vi "findNodes.vi"(0 "reference":refnum<class "Graph.lvclass">, 1 "bounds":T1 {"height" format="%.2f"; "width" format="%.2f"; "y" format="%.2f"; "x" format="%.2f"}, 5 "error in (no error)":errorcluster) -> (14 "reference out":refnum<class "Graph.lvclass">, 15 "FirstNode":refnum<class "AbstractNode.lvclass">, 16 "Nodes":refnum<class "AbstractNode.lvclass">[](array[class]), 17 "AnyFound":bool, 19 "error out":errorcluster)   [LabVIEW 2014, in "Graph.lvclass"]
doc: "Finds a node containing the given point.\n @param p a point\n @return a node containing p or null if no nodes contain p\n */\n public Node findNode(Point2D p)"
uses:
  <resource>/Framework/Providers/Open_GDS/UML/Graph_class/Graph.lvclass
  <resource>/Framework/Providers/Open_GDS/UML/General/Rectangle/Rectangle Rectangle2D.ctl
  <resource>/Framework/Providers/Open_GDS/UML/AbstractNode_class/AbstractNode.lvclass
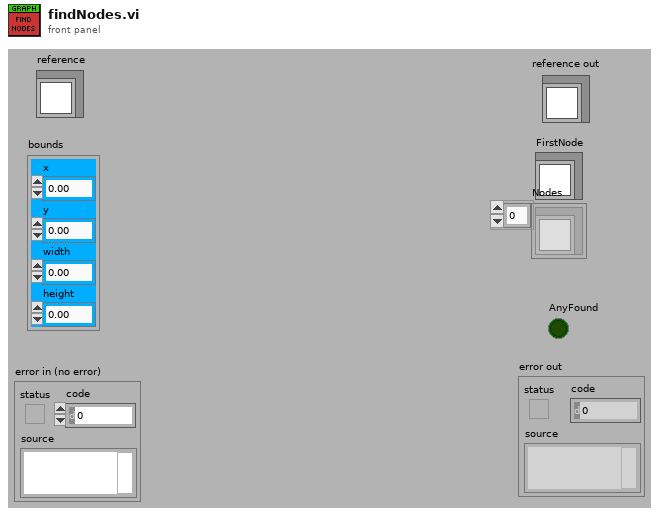
[diagram p1: front panel]
types:
  T1 = typedef "Rectangle Rectangle2D.ctl" = cluster{"x":dbl, "y":dbl, "width":dbl, "height":dbl}
  T2 = typedef "Graph.lvclass/ObjectAttributes.ctl" = cluster{"nodes":refnum<class "AbstractNode.lvclass">[], "edges":refnum<class "AbstractEdge.lvclass">[], "nodesToBeRemoved":refnum<class "AbstractNode.lvclass">[], "edgesToBeRemoved":refnum<class "AbstractEdge.lvclass">[], "needsLayout":bool, "LayoutNodes":refnum<class "AbstractNode.lvclass">[]}
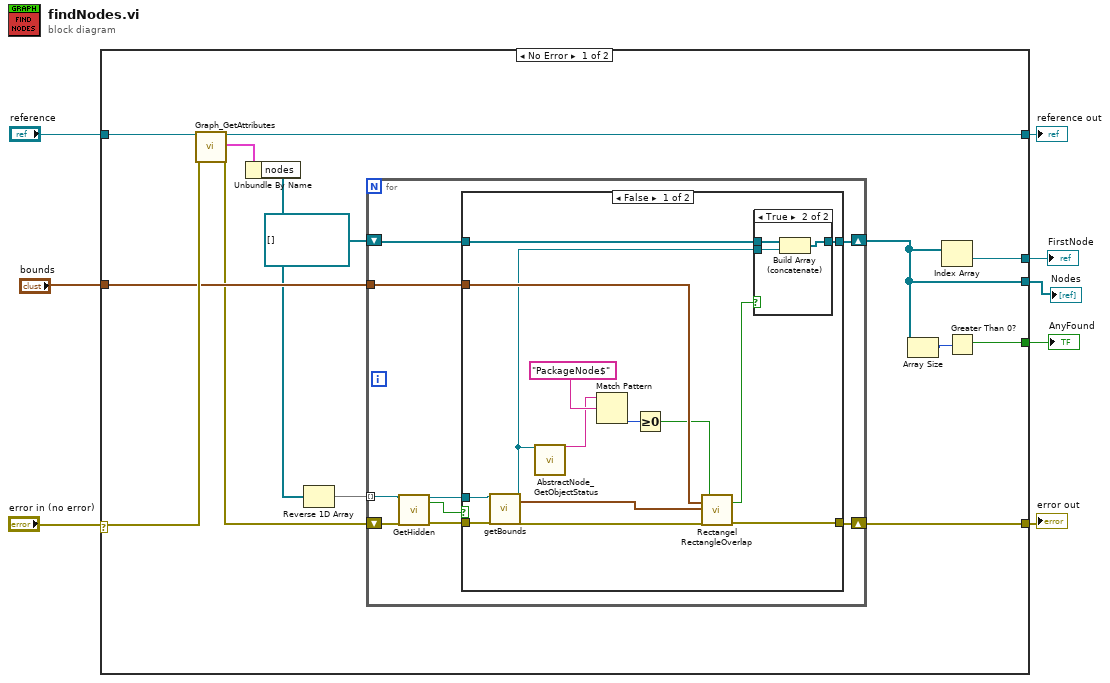
[diagram p0: block diagram]
diagram:
  n1 = case shown="No Error" "error in (no error)" {
    selector: "error in (no error)" -> [w19 w52]
    tunnel: "reference" -> [w22 w53]
    tunnel: [w21 w52] -> w7
    tunnel: [w20 w53] -> w6
    tunnel: "bounds" -> [w18 _]
    tunnel: [w17 _] -> w2
    tunnel: [w16 _] -> w3
    tunnel: [w15 _] -> w1
    frame No Error {
      n2 = call <resource>:"Graph_GetAttributes.vi"("reference in"=w22, "error in (no error)"=w19) -> ("reference out"=w20:refnum<class "Graph.lvclass">, "Data"=w9:T2, "error out"=w13:errorcluster)  [unwired: 1 in, 14 out]
      n3 = Unbundle By Name(w9) -> ("nodes"=w14:refnum<class "AbstractNode.lvclass">[])
      n4 = Reverse 1D Array(array=w14) -> (reversed array=w12:refnum<class "AbstractNode.lvclass">[])
      n5 = for {
        tunnel: w12 -> [w26] mode=indexing
        shift-right: [w30] -> w21
        shift-left: w13 -> [w27]
        tunnel: w18 -> [w31]
        shift-right: [w28] -> w15
        shift-left: refnum<class "AbstractNode.lvclass">[] [] -> [w29]
        n6 = call-dynamic "GetHidden.vi"("reference in"=w26, "error in (no error)"=w27) -> ("reference out"=w25:refnum<class "AbstractNode.lvclass">, "Hidden"=w23:bool, "error out"=w24:errorcluster)  [unwired: 15 in]
        n7 = case shown="False" w23 {
          tunnel: w31 -> [w43 _]
          tunnel: [w41 w51] -> w30
          tunnel: w29 -> [w40 w50]
          tunnel: [w39 w50] -> w28
          tunnel: w25 -> [w38 _]
          tunnel: w24 -> [w37 w51]
          frame False {
            n8 = call-dynamic "getBounds.vi"("reference"=w38, "error in (no error)"=w37) -> ("reference out"=w33:refnum<class "AbstractNode.lvclass">, "bounds"=w44:T1, "error out"=w45:errorcluster)  [unwired: 15 out]
            n9 = call <resource>:"AbstractNode_GetObjectStatus.vi"("reference in"=w33) -> ("Class name"=w32:string)  [unwired: 1 in, 17 out]
            n10 = Match Pattern(string=w32, regular expression="PackageNode$") -> (offset past match=w36:i32)  [unwired: 4 out]
            n11 = Greater Or Equal To 0?(x=w36) -> (x >= 0?=w34:bool)
            n12 = call <resource>:"Rectangel RectangleOverlap.vi"("bounds1"=w43, "bounds2"=w44, "error in (no error)"=w45, "Bound1HasToBeInsideBound2(False)"=w34) -> ("overlap"=w42:bool, "error out"=w41:errorcluster)  [unwired: 14 out]
            n13 = case shown="True" w42 {
              tunnel: w40 -> [w46 w49]
              tunnel: [w46 w48] -> w39
              tunnel: w33 -> [_ w47]
              frame False {
              }
              frame True {
                n14 = Build Array (concatenate)(w49, w47) -> (w48:refnum<class "AbstractNode.lvclass">[])
              }
            }
          }
          frame True {
          }
        }
      }
      n15 = Array Size(array=w15) -> (size(s)=w10:i32)
      n16 = Index Array(array=w15) -> (element=w17:refnum<class "AbstractNode.lvclass">)  [unwired: 1 in]
      n17 = Greater Than 0?(x=w10) -> (x > 0?=w16:bool)
    }
    frame Error {
    }
  }
  "reference out" <- w6
  "error out" <- w7
  "AnyFound" <- w3
  "FirstNode" <- w2
  "Nodes" <- w1
